vi "Filter (G3)-Init.vi"(5 "Filter":T1={"Type"=enum."Lowpass", "CF (kHz)"=0.0, "BW (kHz)"=0.0, "Cascade"=FALSE, "Quadrature"=FALSE, "Scale Factor"=0.0, "Stages"=[], "Class"=enum."Elliptic", "Order"=0, "BWUnits"=enum."Linear"} {"Stages"."IIR Filter"."Forward Coefficients" format="%.4f"; "Stages"."IIR Filter"."Reverse Coefficients" format="%.4f"}, 9 "Sampling rate (Hz)":dbl, 11 "error in (no error)":errorcluster) -> (6 "Filter out":T1={"Type"=enum."Lowpass", "CF (kHz)"=0.0, "BW (kHz)"=0.0, "Cascade"=FALSE, "Quadrature"=FALSE, "Scale Factor"=0.0, "Stages"=[], "Class"=enum."Elliptic", "Order"=0, "BWUnits"=enum."Linear"} {"Stages"."IIR Filter"."Forward Coefficients" format="%.4f"; "Stages"."IIR Filter"."Reverse Coefficients" format="%.4f"}, 15 "error out":errorcluster)   [LabVIEW 2020]
uses:
  XControls/Filter (G3)/Filter Data.ctl
  XControls/Filter (G3)/Filter Type.ctl
  Filter VIs/Filter-Bandwidth Units.ctl
  <vilib>/Analysis/3filter.llb/Filter Passband Type.ctl
  <vilib>/Analysis/NI_AALBase.lvlib
  XControls/Filter (G3)/Filter (G3).xctl
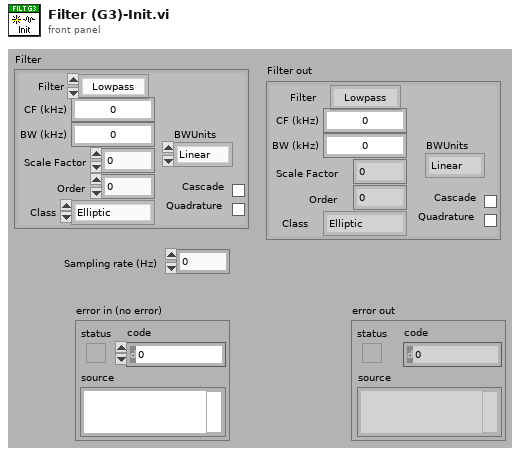
[diagram p1: front panel]
types:
  T1 = typedef "Filter (G3).xctl/Filter Data.ctl" = cluster{"Type":T2, "CF (kHz)":dbl, "BW (kHz)":dbl, "Cascade":bool, "Quadrature":bool, "Scale Factor":dbl, "Stages":cluster{"IIR Filter":cluster{"filter structure":enum32{"IIR 2nd Order", "IIR 4th Order"}, "Reverse Coefficients":dbl[], "Forward Coefficients":dbl[]}, "State":dbl[]}[], "Class":enum16{"Elliptic", "Butterworth"}, "Order":i32, "BWUnits":T3}
  T2 = typedef "Filter (G3).xctl/Filter Type.ctl" = enum16{"OFF", "Lowpass", "Highpass", "Bandpass", "Bandstop"}
  T3 = typedef "Filter-Bandwidth Units.ctl" = enum16{"Linear", "Octaves", "Min-Max"}
  T4 = cluster{"IIR Filter Cluster":cluster{"filter structure":enum32{"IIR 2nd Order", "IIR 4th Order"}, "Reverse Coefficients":dbl[], "Forward Coefficients":dbl[]}, "Final Filter State":dbl[]}[]
  T5 = typedef "NI_AALBase.lvlib/Filter Passband Type.ctl" = enum32{"Lowpass", "Highpass", "Bandpass", "Bandstop"}
  T6 = cluster{"IIR Filter Cluster":cluster{"filter structure":enum32{"IIR 2nd Order", "IIR 4th Order"}, "Reverse Coefficients":dbl[], "Forward Coefficients":dbl[]}, "Final Filter State":dbl[]}
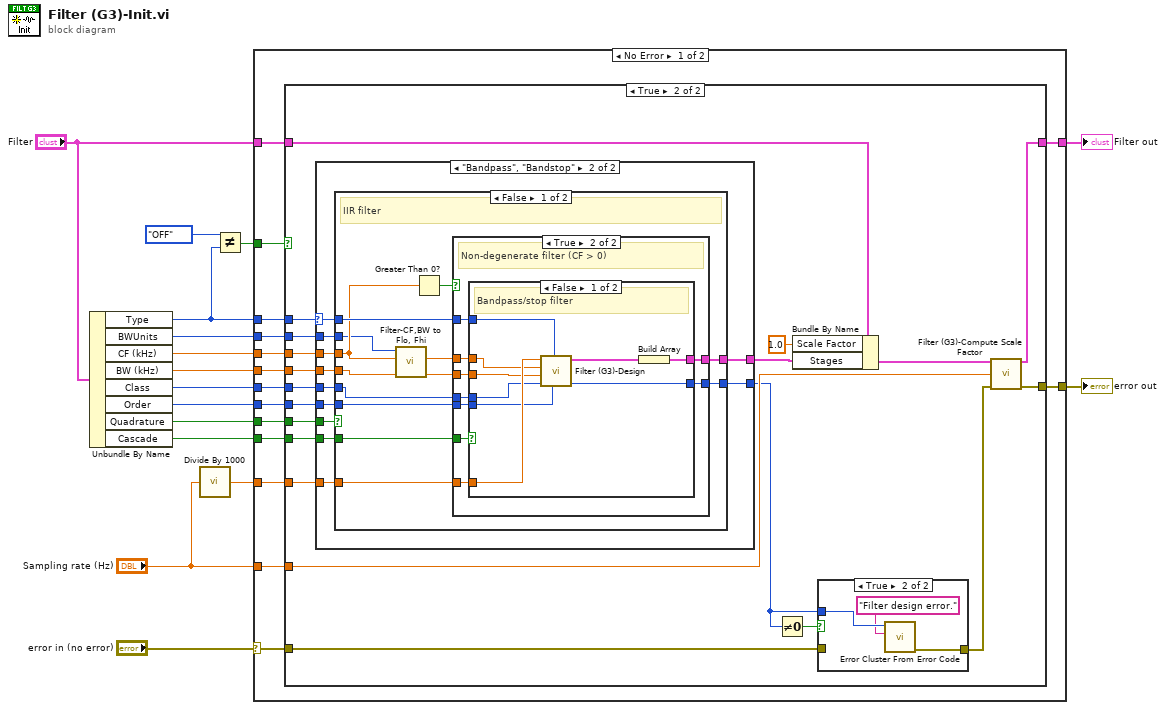
[diagram p0: block diagram]
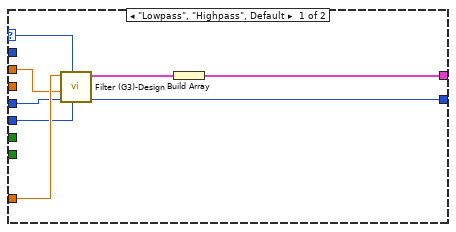
[diagram p4: hidden frame]
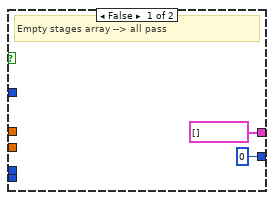
[diagram p5: hidden frame]
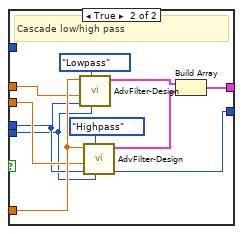
[diagram p6: hidden frame]
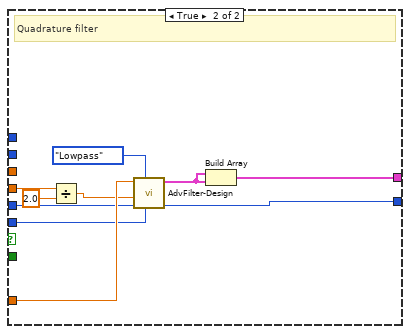
[diagram p7: hidden frame]
diagram:
  n1 = Unbundle By Name("Filter") -> ("Type"=w3:T2, "BWUnits"=w2:T3, "CF (kHz)"=w13:dbl, "BW (kHz)"=w12:dbl, "Class"=w8:enum16{"Elliptic", "Butterworth"}, "Order"=w7:i32, "Quadrature"=w10:bool, "Cascade"=w6:bool)
  n2 = call "Divide By 1000.vi"("X"="Sampling rate (Hz)") -> ("X/1000"=w4:dbl)
  n3 = Not Equal?(x=Filter_Type."OFF" ("Type"), y=w3) -> (x != y?=w9:bool)
  n4 = case shown="No Error" "error in (no error)" {
    selector: "error in (no error)" -> [w24 w131]
    tunnel: w9 -> [w31 _]
    tunnel: w3 -> [w30 _]
    tunnel: "Sampling rate (Hz)" -> [w29 _]
    tunnel: "Filter" -> [w28 w132]
    tunnel: [w27 w132] -> w14
    tunnel: w13 -> [w26 _]
    tunnel: w12 -> [w25 _]
    tunnel: [w23 w131] -> w11
    tunnel: w10 -> [w22 _]
    tunnel: w8 -> [w21 _]
    tunnel: w7 -> [w20 _]
    tunnel: w4 -> [w19 _]
    tunnel: w6 -> [w18 _]
    tunnel: w2 -> [w17 _]
    frame No Error {
      n5 = case shown="True" w31 {
        tunnel: w30 -> [_ w47]
        tunnel: w29 -> [_ w48]
        tunnel: w28 -> [w33 w53]
        tunnel: [w33 w38] -> w27
        tunnel: w26 -> [_ w52]
        tunnel: w25 -> [_ w51]
        tunnel: w24 -> [w32 w49]
        tunnel: [w32 w35] -> w23
        tunnel: w22 -> [_ w46]
        tunnel: w21 -> [_ w45]
        tunnel: w20 -> [_ w44]
        tunnel: w19 -> [_ w42]
        tunnel: w18 -> [_ w40]
        tunnel: w17 -> [_ w34]
        frame False {
        }
        frame True {
          n6 = case shown="\"Bandpass\", \"Bandstop\"" w47 {
            selector: w47 -> [w58 w67]
            tunnel: w52 -> [w59 w75]
            tunnel: w51 -> [_ w76]
            tunnel: w46 -> [_ w74]
            tunnel: w45 -> [w64 w71]
            tunnel: w44 -> [w63 w72]
            tunnel: [w61 w69] -> w43
            tunnel: w42 -> [w65 w73]
            tunnel: [w60 w70] -> w41
            tunnel: w40 -> [_ w68]
            tunnel: w34 -> [_ w66]
            frame "Lowpass", "Highpass", Default {
              n7 = call "Filter (G3)-Design.vi"("order"=w63, "Type"=w58, "Class"=w64, "low cutoff freq: fl"=w59, "sampling freq: fs"=w65) -> ("error"=w60:i32, "IIR Filter"=w62:T6)  [unwired: 5 in]
              n8 = Build Array(w62) -> (w61:T4)
            }
            frame "Bandpass", "Bandstop" {
              n9 = case shown="False" w74 {
                tunnel: w76 -> [w79 w130]
                tunnel: w75 -> [w82 _]
                tunnel: w73 -> [w87 w127]
                tunnel: w72 -> [w86 w126]
                tunnel: w71 -> [w85 w125]
                tunnel: [w83 w123] -> w70
                tunnel: [w84 w121] -> w69
                tunnel: w68 -> [w89 _]
                tunnel: w67 -> [w88 _]
                tunnel: w66 -> [w80 _]
                frame False {
                  # "IIR filter"
                  n10 = call "Filter-CF,BW to Flo, Fhi.vi"("BW"=w79, "CF (kHz)"=w82, "BWUnits"=w80) -> ("Fmin"=w77:dbl, "Fmax"=w78:dbl)  [unwired: 7 in]
                  n11 = Greater Than 0?(x=w82) -> (x > 0?=w81:bool)
                  n12 = case shown="True" w81 {
                    tunnel: w89 -> [_ w100]
                    tunnel: w88 -> [_ w99]
                    tunnel: w87 -> [_ w98]
                    tunnel: w78 -> [_ w97]
                    tunnel: w77 -> [_ w96]
                    tunnel: w86 -> [_ w95]
                    tunnel: w85 -> [_ w94]
                    tunnel: [T4 [] w93] -> w84
                    tunnel: [0 ("error") w92] -> w83
                    frame False {
                      # "Empty stages array --> all pass"
                    }
                    frame True {
                      # "Non-degenerate filter (CF > 0)"
                      n13 = case shown="False" w100 {
                        tunnel: w99 -> [w109 _]
                        tunnel: w98 -> [w108 w120]
                        tunnel: w97 -> [w107 w119]
                        tunnel: w96 -> [w106 w118]
                        tunnel: w95 -> [w105 w110]
                        tunnel: w94 -> [w104 w111]
                        tunnel: [w103 w114] -> w93
                        tunnel: [w101 w112] -> w92
                        frame False {
                          # "Bandpass/stop filter"
                          n14 = call "Filter (G3)-Design.vi"("order"=w105, "Type"=w109, "Class"=w104, "low cutoff freq: fl"=w106, "high cutoff freq: fh"=w107, "sampling freq: fs"=w108) -> ("error"=w101:i32, "IIR Filter"=w102:T6)  [unwired: 4 in]
                          n15 = Build Array(w102) -> (w103:T4)
                        }
                        frame True {
                          # "Cascade low/high pass"
                          n16 = call "AdvFilter-Design.vi"("order"=w110, "filter type"=Filter_Passband_Type."Lowpass", "Class"=w111, "low cutoff freq: fl"=w119, "sampling freq: fs"=w120) -> ("IIR Filter"=w115:T6)  [unwired: 5 in, 1 out]
                          n17 = call "AdvFilter-Design.vi"("order"=w110, "filter type"=Filter_Passband_Type."Highpass", "Class"=w111, "low cutoff freq: fl"=w118, "sampling freq: fs"=w120) -> ("error"=w112:i32, "IIR Filter"=w113:T6)  [unwired: 5 in]
                          n18 = Build Array(w115, w113) -> (w114:T4)
                        }
                      }
                    }
                  }
                }
                frame True {
                  # "Quadrature filter"
                  n19 = Divide(x=w130, y=2.0) -> (x/y=w124:dbl)
                  n20 = call "AdvFilter-Design.vi"("order"=w126, "filter type"=Filter_Passband_Type."Lowpass", "Class"=w125, "low cutoff freq: fl"=w124, "sampling freq: fs"=w127) -> ("error"=w123:i32, "IIR Filter"=w122:T6)  [unwired: 5 in]
                  n21 = Build Array(w122, w122) -> (w121:T4)
                }
              }
            }
          }
          n22 = Not Equal To 0?(x=w41) -> (x != 0?=w50:bool)
          n23 = Bundle By Name(cluster=w53, "Scale Factor"=1.0, "Stages"=w43) -> (w39:T1)
          n24 = case shown="True" w50 {
            tunnel: [w54 w56] -> w36
            tunnel: w49 -> [w54 _]
            tunnel: w41 -> [_ w57]
            frame False {
            }
            frame True {
              n25 = call <vilib>:"Error Cluster From Error Code.vi"("error message (\"\")"="Filter design error." ("error message (\"\")"), "error code (0)"=w57) -> ("error out"=w56:errorcluster)  [unwired: 7 in]
            }
          }
          n26 = call "Filter (G3)-Compute Scale Factor.vi"("Filter"=w39, "Sampling Rate (Hz)"=w48, "error in (no error)"=w36) -> ("Filter out"=w38:T1, "error out"=w35:errorcluster)  [unwired: 11 in]
        }
      }
    }
    frame Error {
    }
  }
  "error out" <- w11
  "Filter out" <- w14
